vi "Stop Core.vi"(10 "final error code":i32, 11 "_Parent Actor Template in":refnum<class "_Parent Actor Template.lvclass">) -> (3 "_Parent Actor Template out":refnum<class "_Parent Actor Template.lvclass">)   [LabVIEW 2016, in "_Parent Actor Template.lvlib" / "_Parent Actor Template.lvclass"]
doc: "(<B>Filename</B>: Actor Framework.lvlib:Actor.lvclass:Stop Core.vi)\n\nDefines what the actor does before it stops. Use the <B>final error code</B> input to determine whether the actor shut down in response to an error.\n\nBy default, this method does nothing. A descendant class may override it to define behavior, such as shutting down any processes the actor initiated in its override of the Actor Core method."
uses:
  _Parent Actor Template.lvclass
  <vilib>/ActorFramework/Actor/Actor.lvclass
  Enum - Debug Context.ctl
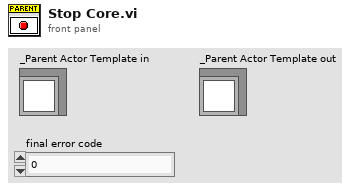
[diagram p1: front panel]
types:
  T1 = typedef "_Parent Actor Template.lvlib/_Parent Actor Template.lvclass/Enum - Debug Context.ctl" = enum16{"Null", "Startup", "Shutdown"}
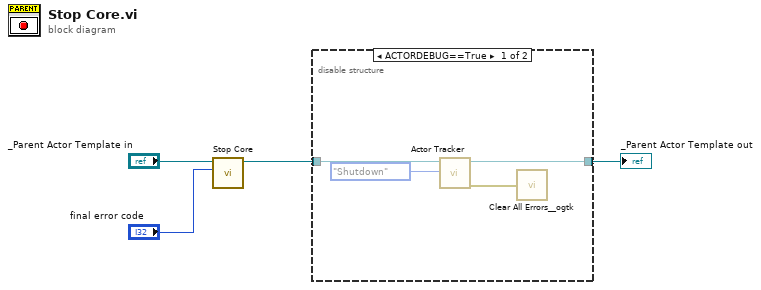
[diagram p0: block diagram]
diagram:
  n1 = call-parent "Stop Core.vi"("final error code"="final error code", "Actor in"="_Parent Actor Template in") -> ("Actor out"=w2:refnum<class "_Parent Actor Template.lvclass">)  [unwired: 9 in]
  n2 = disable-structure shown="ACTORDEBUG==True" {
    disable-tunnel: w2 -> [w8 w9]
    disable-tunnel: [w7 w9] -> w1
    frame condition #0 {
      n3 = call "Actor Tracker.vi"("Context"=Enum_-_Debug_Context."Shutdown", "_Parent Actor Template in"=w8) -> ("error out"=w6:errorcluster, "_Parent Actor Template out"=w7:refnum<class "_Parent Actor Template.lvclass">)  [unwired: 8 in]
      n4 = call <userlib>:"Clear All Errors__ogtk.vi"("Error In"=w6) -> ()  [unwired: 3 in, 1 out]
    }
    frame condition #1 (active) {
    }
  }
  "_Parent Actor Template out" <- w1
